vi "User Retrieve Record.vi"(8 "error in (no error)":errorcluster, 11 "Statement Refnum":T1) -> (0 "error out":errorcluster, 2 "User Record":T2, 3 "Statement Refnum":T1)   [LabVIEW 2011]
uses:
  User Record.ctl
  Summitek EXT/ODBC/SQL Controls/Statement Refnum.ctl
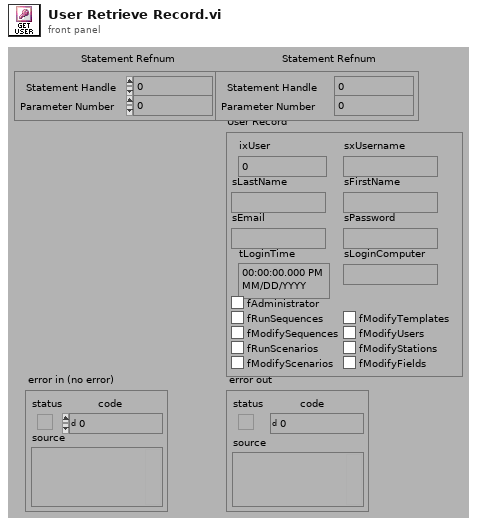
[diagram p1: front panel]
types:
  T1 = typedef "Statement Refnum.ctl" = cluster{"Statement Handle":i32, "Parameter Number":u16}
  T2 = typedef "User Record.ctl" = cluster{"ixUser":i32, "sxUsername":string, "sLastName":string, "sFirstName":string, "sEmail":string, "sPassword":string, "tLoginTime":timestamp, "sLoginComputer":string, "fAdministrator":bool, "fRunSequences":bool, "fModifySequences":bool, "fRunScenarios":bool, "fModifyScenarios":bool, "fModifyTemplates":bool, "fModifyUsers":bool, "fModifyStations":bool, "fModifyFields":bool}
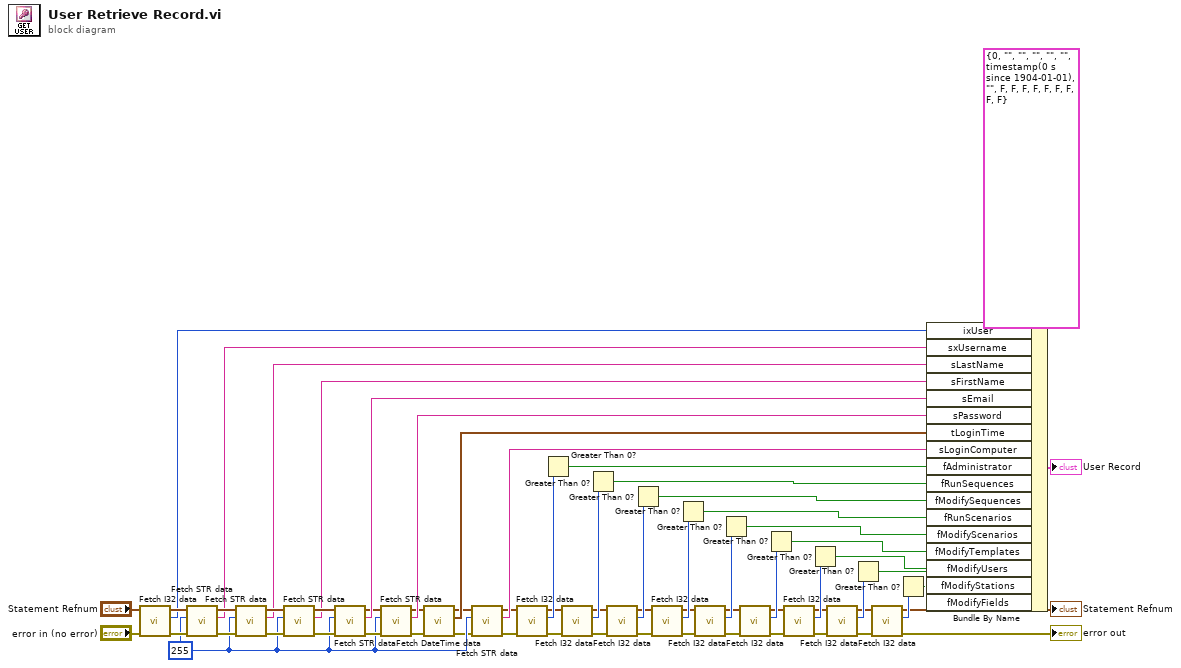
[diagram p0: block diagram]
diagram:
  w46 = 255 ("Buffer Size")
  n1 = call "Fetch I32 data.vi"("error in (no error)"="error in (no error)", "Statement Refnum"="Statement Refnum") -> ("error out"=w60:errorcluster, "Data"=w58:i32, "Statement Refnum"=w59:T1)  [unwired: 3 out]
  n2 = call "Fetch STR data.vi"("error in (no error)"=w60, "Buffer Size"=w46, "Statement Refnum"=w59) -> ("error out"=w62:errorcluster, "Data"=w51:string, "Statement Refnum"=w61:T1)  [unwired: 2 out]
  n3 = call "Fetch STR data.vi"("error in (no error)"=w62, "Buffer Size"=w46, "Statement Refnum"=w61) -> ("error out"=w57:errorcluster, "Data"=w53:string, "Statement Refnum"=w56:T1)  [unwired: 2 out]
  n4 = call "Fetch STR data.vi"("error in (no error)"=w57, "Buffer Size"=w46, "Statement Refnum"=w56) -> ("error out"=w54:errorcluster, "Data"=w52:string, "Statement Refnum"=w55:T1)  [unwired: 2 out]
  n5 = call "Fetch STR data.vi"("error in (no error)"=w54, "Buffer Size"=w46, "Statement Refnum"=w55) -> ("error out"=w47:errorcluster, "Data"=w50:string, "Statement Refnum"=w48:T1)  [unwired: 2 out]
  n6 = call "Fetch STR data.vi"("error in (no error)"=w47, "Buffer Size"=w46, "Statement Refnum"=w48) -> ("error out"=w44:errorcluster, "Data"=w45:string, "Statement Refnum"=w43:T1)  [unwired: 2 out]
  n7 = call "Fetch DateTime data.vi"("error in (no error)"=w44, "Statement Refnum"=w43) -> ("error out"=w40:errorcluster, "Data"=w42:timestamp, "Statement Refnum"=w41:T1)  [unwired: 3 out]
  n8 = call "Fetch STR data.vi"("error in (no error)"=w40, "Buffer Size"=w46, "Statement Refnum"=w41) -> ("error out"=w29:errorcluster, "Data"=w39:string, "Statement Refnum"=w30:T1)  [unwired: 2 out]
  n9 = call "Fetch I32 data.vi"("error in (no error)"=w29, "Statement Refnum"=w30) -> ("error out"=w28:errorcluster, "Data"=w38:i32, "Statement Refnum"=w17:T1)  [unwired: 3 out]
  n10 = Greater Than 0?(x=w38) -> (x > 0?=w31:bool)
  n11 = call "Fetch I32 data.vi"("error in (no error)"=w28, "Statement Refnum"=w17) -> ("error out"=w27:errorcluster, "Data"=w37:i32, "Statement Refnum"=w18:T1)  [unwired: 3 out]
  n12 = Greater Than 0?(x=w37) -> (x > 0?=w16:bool)
  n13 = call "Fetch I32 data.vi"("error in (no error)"=w27, "Statement Refnum"=w18) -> ("error out"=w26:errorcluster, "Data"=w36:i32, "Statement Refnum"=w19:T1)  [unwired: 3 out]
  n14 = Greater Than 0?(x=w36) -> (x > 0?=w15:bool)
  n15 = call "Fetch I32 data.vi"("error in (no error)"=w26, "Statement Refnum"=w19) -> ("error out"=w25:errorcluster, "Data"=w35:i32, "Statement Refnum"=w20:T1)  [unwired: 3 out]
  n16 = Greater Than 0?(x=w35) -> (x > 0?=w14:bool)
  n17 = call "Fetch I32 data.vi"("error in (no error)"=w25, "Statement Refnum"=w20) -> ("error out"=w24:errorcluster, "Data"=w34:i32, "Statement Refnum"=w21:T1)  [unwired: 3 out]
  n18 = Greater Than 0?(x=w34) -> (x > 0?=w13:bool)
  n19 = call "Fetch I32 data.vi"("error in (no error)"=w24, "Statement Refnum"=w21) -> ("error out"=w23:errorcluster, "Data"=w33:i32, "Statement Refnum"=w22:T1)  [unwired: 3 out]
  n20 = Greater Than 0?(x=w33) -> (x > 0?=w12:bool)
  n21 = call "Fetch I32 data.vi"("error in (no error)"=w23, "Statement Refnum"=w22) -> ("error out"=w5:errorcluster, "Data"=w32:i32, "Statement Refnum"=w6:T1)  [unwired: 3 out]
  n22 = Greater Than 0?(x=w32) -> (x > 0?=w11:bool)
  n23 = call "Fetch I32 data.vi"("error in (no error)"=w5, "Statement Refnum"=w6) -> ("error out"=w4:errorcluster, "Data"=w10:i32, "Statement Refnum"=w3:T1)  [unwired: 3 out]
  n24 = Greater Than 0?(x=w10) -> (x > 0?=w8:bool)
  n25 = call "Fetch I32 data.vi"("error in (no error)"=w4, "Statement Refnum"=w3) -> ("error out"=→"error out":errorcluster, "Data"=w9:i32, "Statement Refnum"=→"Statement Refnum":T1)  [unwired: 3 out]
  n26 = Greater Than 0?(x=w9) -> (x > 0?=w7:bool)
  n27 = Bundle By Name(cluster=T2 {"ixUser"=0, "sxUsername"="", "sLastName"="", "sFirstName"="", "sEmail"="", "sPassword"="", "tLoginTime"=timestamp(0 s since 1904-01-01), "sLoginComputer"="", "fAdministrator"=FALSE, "fRunSequences"=FALSE, "fModifySequences"=FALSE, "fRunScenarios"=FALSE, "fModifyScenarios"=FALSE, "fModifyTemplates"=FALSE, "fModifyUsers"=FALSE, "fModifyStations"=FALSE, "fModifyFields"=FALSE} ("User Information"), "ixUser"=w58, "sxUsername"=w51, "sLastName"=w53, "sFirstName"=w52, "sEmail"=w50, "sPassword"=w45, "tLoginTime"=w42, "sLoginComputer"=w39, "fAdministrator"=w31, "fRunSequences"=w16, "fModifySequences"=w15, "fRunScenarios"=w14, "fModifyScenarios"=w13, "fModifyTemplates"=w12, "fModifyUsers"=w11, "fModifyStations"=w8, "fModifyFields"=w7) -> (→"User Record":T2)
